vi "Send Request.vi"(5 "Target Task":u32, 6 "Timeout mS (5000)":i32=5000, 7 "Target Node":u32, 8 "error in (no error)":errorcluster, 9 "Type":string, 10 "Payload":u8[](array[numeric]), 11 "TCPMessageAPI in":refnum<class "TCPMessageAPI.lvclass">) -> (0 "error out":errorcluster, 2 "Reply":T1, 3 "TCPMessageAPI out":refnum<class "TCPMessageAPI.lvclass">)   [LabVIEW 2020, in "Vecto.lvlib" / "TCPMessageAPI.lvclass"]
uses:
  TCPMessageAPI.lvclass
  TCPMessageAPI.lvclass/TCPMessageAPI.ctl
  lv-promises/Promises/Future/Future.lvclass
  lv-promises/Promises/Promise/Promise.lvclass
  ReplyValue/ReplyValue.lvclass
  proto/TcpPayload/Data.ctl
  proto/TcpPayload/TcpPayload.lvlib
  Send Message Data.ctl
  Vecto.lvlib
  TCPMessaging/TCPMessaging.lvclass
  C:/dev/lv20CE/relink/lv-promises/Promises/Value/Value.lvclass
  C:/dev/lv20CE/relink/lv-vecto/Vecto/ReplyValue/ReplyValue.lvclass
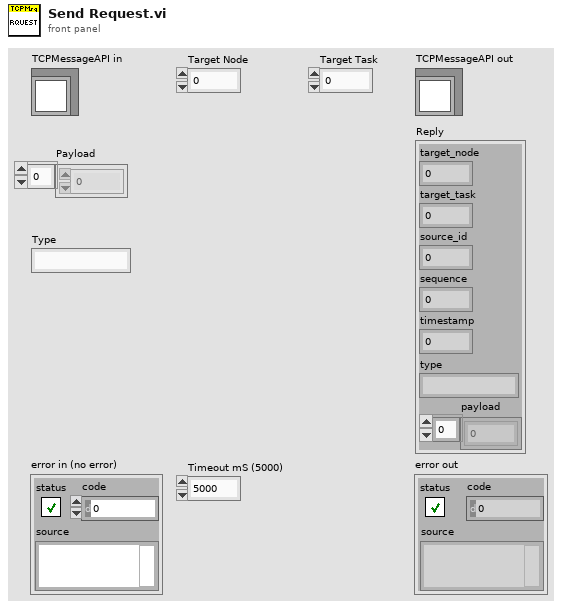
[diagram p1: front panel]
types:
  T1 = typedef "TcpPayload.lvlib/Data.ctl" = cluster{"target_node":u32, "target_task":u32, "source_id":u32, "sequence":u32, "timestamp":u64, "type":string, "payload":u8[]}
  T2 = typedef "Vecto.lvlib/Send Message Data.ctl" = cluster{"TcpPayload":T1, "Register Reply":bool, "Reply Promise":refnum<class "Promise.lvclass">, "Reply Deadline":dbl}
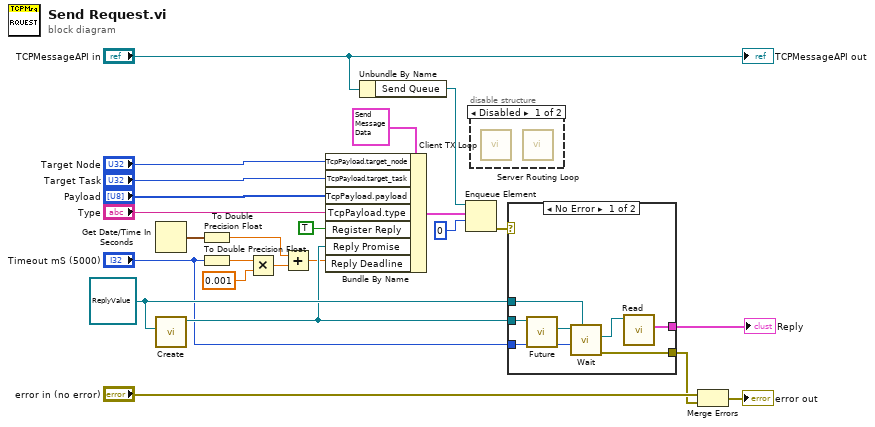
[diagram p0: block diagram]
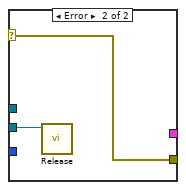
[diagram p3: hidden frame]
diagram:
  w13 = refnum<class "ReplyValue.lvclass"> refnum ("Vecto.lvlib:ReplyValue.lvclass")
  n1 = Get Date/Time In Seconds() -> (seconds since 1Jan1904=w5:timestamp)
  n2 = call "Create.vi"("Result Type"=w13) -> ("Promise"=w11:refnum<class "Promise.lvclass">)  [unwired: 9 in, 1 out]
  n3 = To Double Precision Float(number=w5) -> (double precision float=w4:dbl)
  n4 = To Double Precision Float(number="Timeout mS (5000)") -> (double precision float=w7:dbl)
  n5 = Multiply(x=w7, y=0.001) -> (x*y=w3:dbl)
  n6 = Add(x=w4, y=w3) -> (x+y=w2:dbl)
  n7 = Bundle By Name(cluster=T2 {"TcpPayload"={"target_node"=0, "target_task"=0, "source_id"=0, "sequence"=0, "timestamp"=0, "type"="", "payload"=[]}, "Register Reply"=FALSE, "Reply Promise"=refnum, "Reply Deadline"=0.0} ("Send Message Data"), "TcpPayload.target_node"="Target Node", "TcpPayload.target_task"="Target Task", "TcpPayload.payload"="Payload", "TcpPayload.type"="Type", "Register Reply"=TRUE, "Reply Promise"=w11, "Reply Deadline"=w2) -> (w1:T2)
  n8 = Unbundle By Name("TCPMessageAPI in") -> ("Send Queue"=w16:refnum<queue>)
  n9 = Enqueue Element(queue=w16, element=w1, timeout in ms (-1)=0) -> (error out=w14:errorcluster)  [unwired: 1 in, 2 out]
  n10 = disable-structure shown="Disabled" {
    frame Disabled {
      n11 = call "Client TX Loop.vi"() -> ()  [unwired: 11 in, 1 out]
      n12 = call "Server Routing Loop.vi"() -> ()  [unwired: 11 in, 1 out]
    }
    frame Enabled {
    }
  }
  n13 = case shown="No Error" w14 {
    selector: w14 -> [_ w32]
    tunnel: w13 -> [w31 _]
    tunnel: "Timeout mS (5000)" -> [w30 _]
    tunnel: w11 -> [w25 w33]
    tunnel: [w28 _] -> w12
    tunnel: [w27 w32] -> w9
    frame No Error {
      n14 = call "Future.vi"("Promise in"=w25) -> ("Future"=w26:refnum<class "Future.lvclass">)  [unwired: 9 in, 1 out]
      n15 = call "Wait.vi"("Result Type"=w31, "Timeout mS (-1)"=w30, "Future in"=w26) -> ("error out"=w27:errorcluster, "Result"=w29:refnum<class "ReplyValue.lvclass">)  [unwired: 7 in]
      n16 = call "Read.vi"("ReplyValue in"=w29) -> ("TcpPayload"=w28:T1)  [unwired: 10 in]
    }
    frame Error {
      n17 = call "Release.vi"("Promise in"=w33) -> ()  [unwired: 11 in]
    }
  }
  "Reply" <- w12
  n18 = Merge Errors("error in (no error)", w9) -> (→"error out":errorcluster)
  "TCPMessageAPI out" <- "TCPMessageAPI in"
